vi "DAQ Loop.vi"(7 "DAQ Exit":refnum<notifier>, 8 "error in":errorcluster, 10 "DAQ Queue":refnum<queue>, 11 "PLC Queue":refnum<queue>) -> (0 "error out":errorcluster)   [LabVIEW 2014, in "DAQ.lvlib"]
uses:
  DAQ.lvlib
  support/Message Queue/Message Queue.lvlib
  <vilib>/Utility/error.llb/Error Cluster From Error Code.vi
  support/Message Queue/Enqueue Message (Single).vi
  TypeDefs/DAQ data.ctl
  <vilib>/ErrorRing/Error Ring.xnode
  support/Message Queue/Message Cluster.ctl
panel:
  out "DAQ message":string
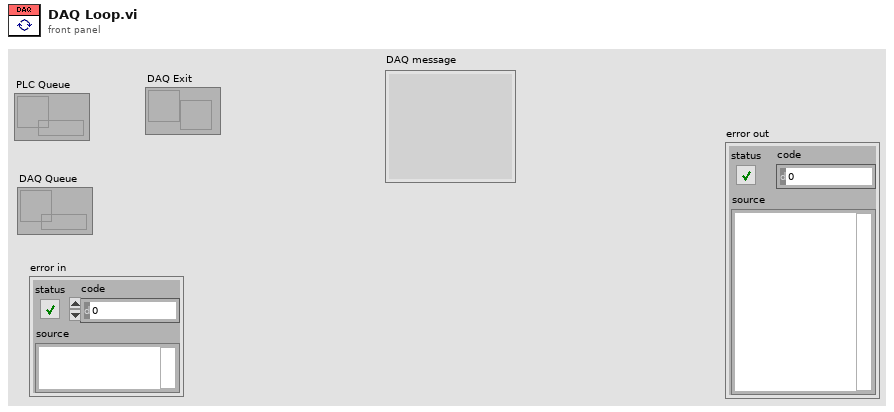
[diagram p1: front panel]
types:
  T1 = typedef "DAQ.lvlib/DAQ data.ctl" = cluster{"Power switch (DI)":cluster{"Channel":tag, "Data":bool}, "Dispose barrel (DI)":cluster{"Channel":tag, "Data":bool}, "Pump status (DO)":cluster{"Channel":tag, "Data":bool}, "Barrel position (AI)":cluster{"Channel":tag, "Data":dbl}}
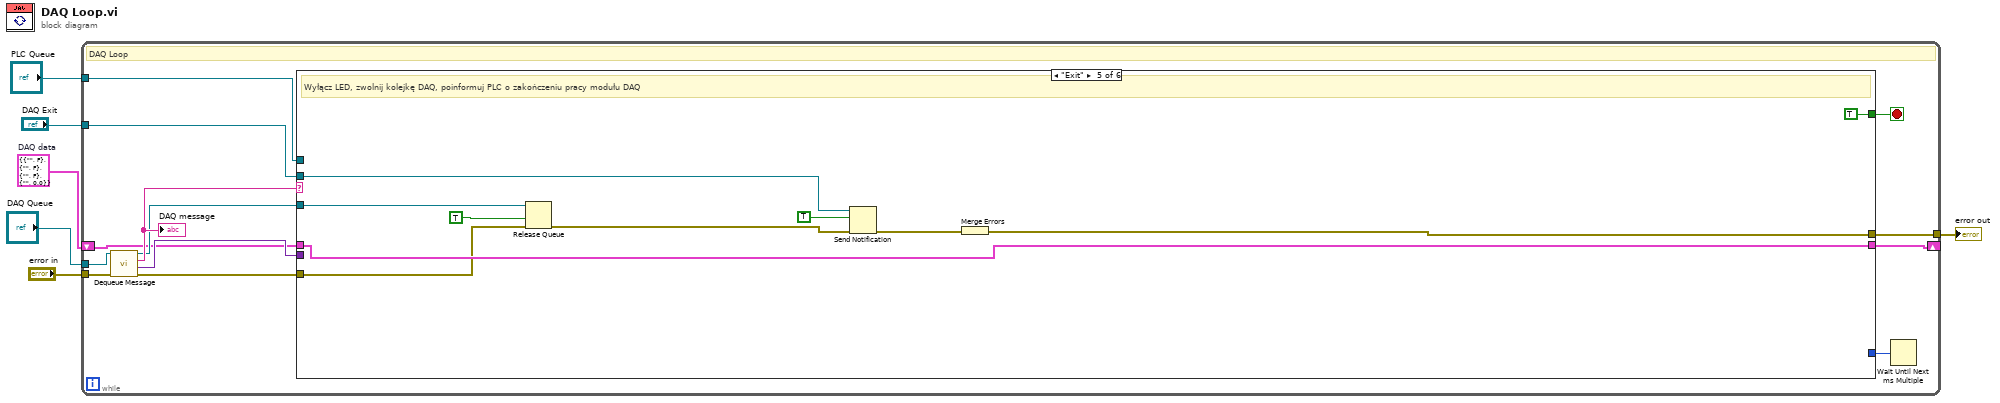
[diagram p0: block diagram]
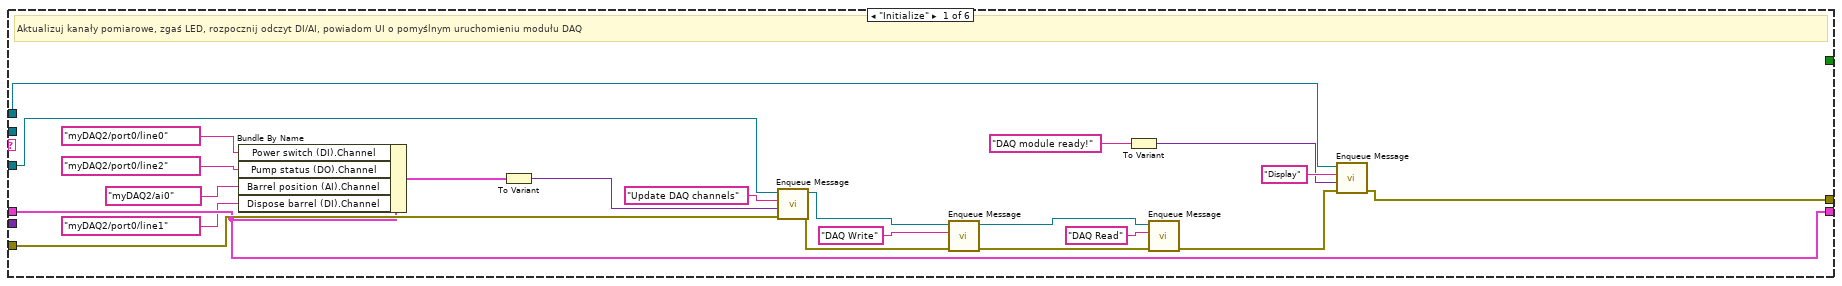
[diagram p2: hidden frame]
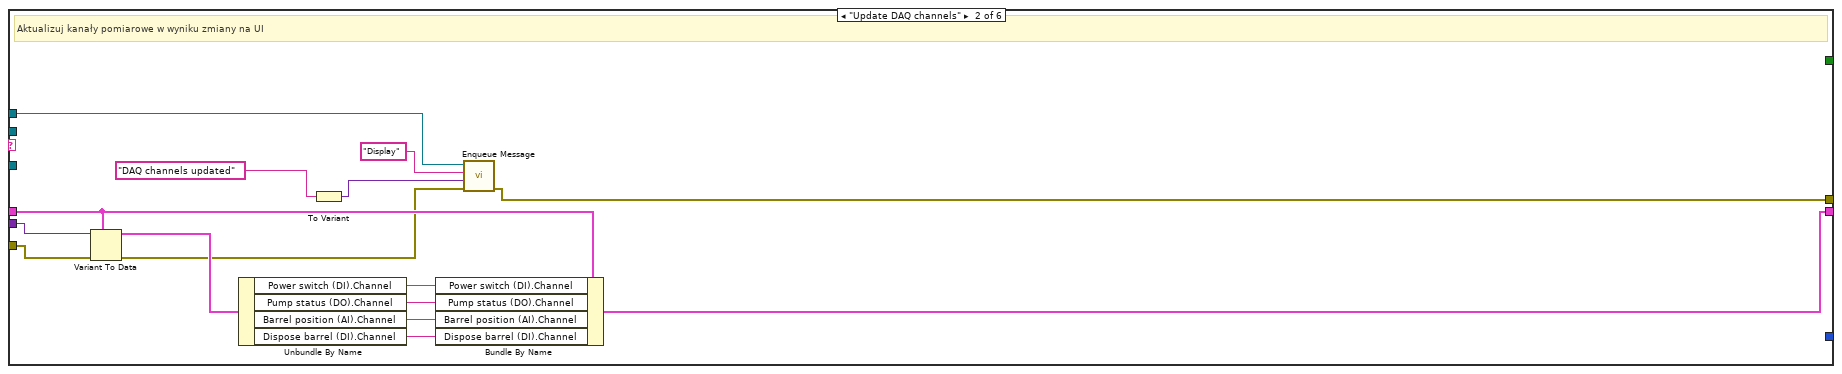
[diagram p3: hidden frame]
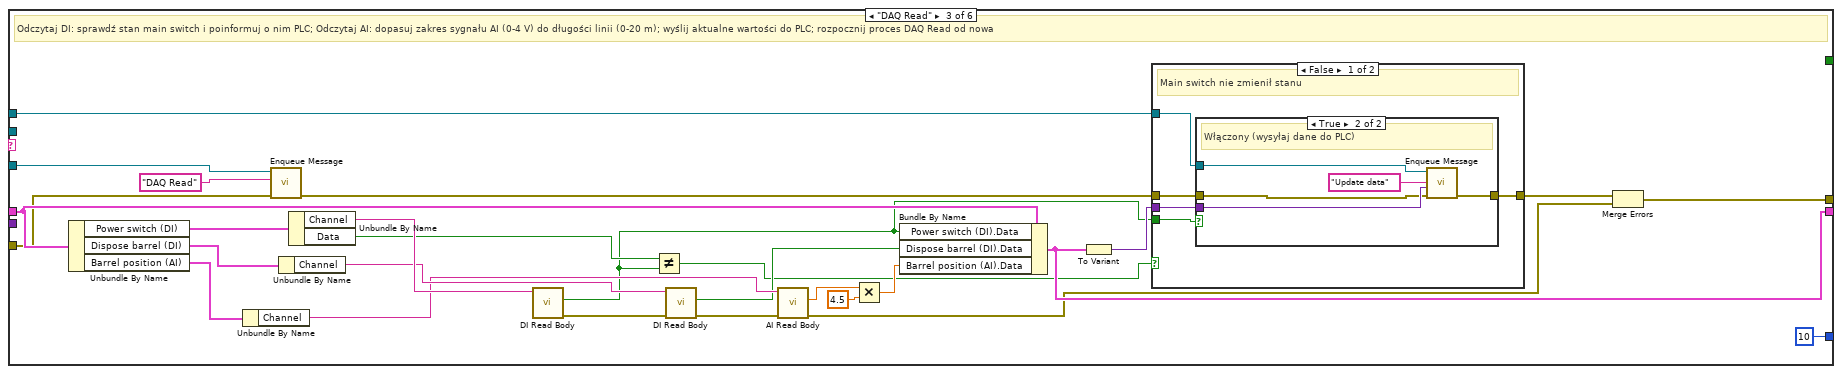
[diagram p4: hidden frame]
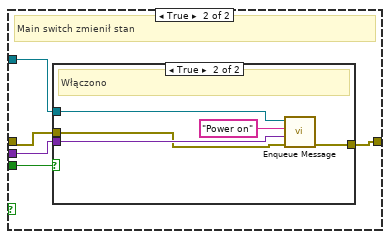
[diagram p6: hidden frame]
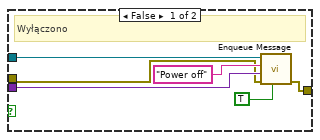
[diagram p7: hidden frame]
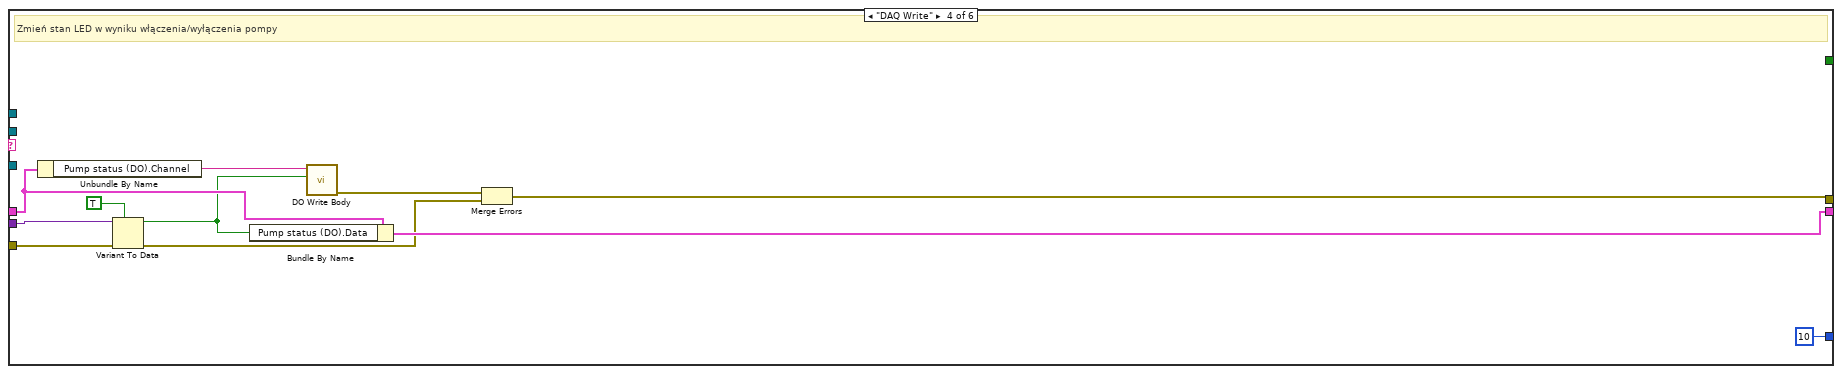
[diagram p8: hidden frame]
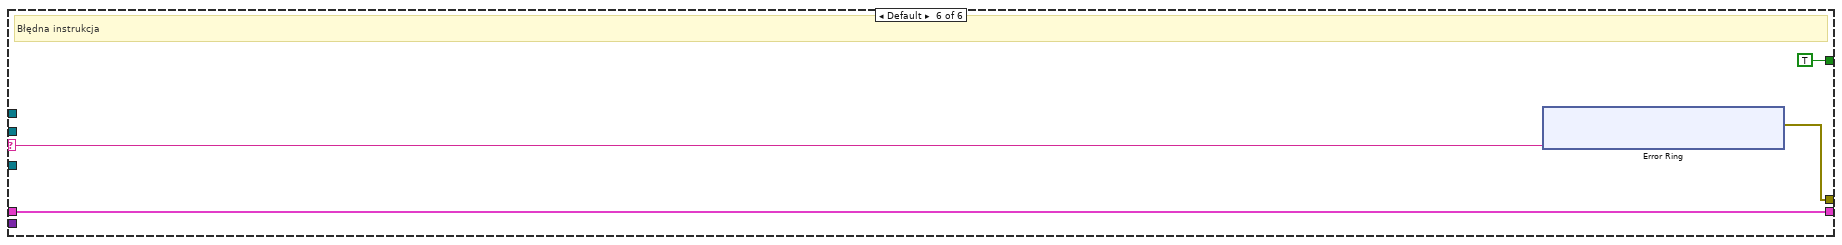
[diagram p9: hidden frame]
diagram:
  w5 = T1 {"Power switch (DI)"={"Channel"="", "Data"=FALSE}, "Dispose barrel (DI)"={"Channel"="", "Data"=FALSE}, "Pump status (DO)"={"Channel"="", "Data"=FALSE}, "Barrel position (AI)"={"Channel"="", "Data"=0.0}}  # DAQ data
  n1 = while {
    tunnel: "error in" -> [w18]
    tunnel: "DAQ Queue" -> [w13]
    tunnel: [w16] -> w2
    tunnel: "PLC Queue" -> [w12]
    tunnel: "DAQ Exit" -> [w10]
    shift-right: [w8] -> _
    shift-left: w5 -> [w9]
    stop <- w14 stop-if-true
    # "DAQ Loop"
    n2 = call "Dequeue Message.vi"("error in (no error)"=w18, "Message Queue"=w13) -> ("error out"=w17:errorcluster, "Message Data"=w15:variant, "Message"=w19:string, "dup Message Queue"=w11:refnum<queue>)  [unwired: 6 in]
    "DAQ message" <- w19
    n3 = case shown="\"Exit\"" w19 {
      selector: w19 -> [_ _ _ _ _ w133]
      tunnel: w17 -> [w38 w55 w60 w120 w123 _]
      tunnel: [w35 w45 w57 w111 w122 w132] -> w16
      tunnel: w15 -> [_ w56 _ w119 _ _]
      tunnel: w12 -> [w39 w44 w65 _ _ _]
      tunnel: [_ _ _ _ TRUE TRUE] -> w14
      tunnel: w11 -> [w37 _ w77 _ w131 _]
      tunnel: w10 -> [_ _ _ _ w130 _]
      tunnel: w9 -> [w27 w53 w78 w116 w125 w134]
      tunnel: [w27 w48 w68 w118 w125 w134] -> w8
      tunnel: [_ _ u32 10 ("millisecond multiple") u32 10 ("millisecond multiple") _ _] -> w7
      frame "Initialize" {
        # "Aktualizuj kanały pomiarowe, zgaś LED, rozpocznij odczyt DI/AI, powiadom UI o pomyślnym uruchomieniu modułu DAQ"
        n4 = Bundle By Name(cluster=w27, "Power switch (DI).Channel"=tag "myDAQ2/port0/line0", "Pump status (DO).Channel"=tag "myDAQ2/port0/line2" ("Power switch (DI).Channel"), "Barrel position (AI).Channel"=tag "myDAQ2/ai0", "Dispose barrel (DI).Channel"=tag "myDAQ2/port0/line1" ("Power switch (DI).Channel")) -> (w26:T1)
        n5 = To Variant(anything=w26) -> (Variant=w25:variant)
        n6 = call-poly "Enqueue Message.vi"("error in (no error)"=w38, "Message Data"=w25, "Message"="Update DAQ channels", "Message Queue"=w37) -> ("error out"=w32:errorcluster, "dup Message Queue"=w31:refnum<queue>)  [unwired: 6 in]
        n7 = call-poly "Enqueue Message.vi"("error in (no error)"=w32, "Message"="DAQ Write", "Message Queue"=w31) -> ("error out"=w29:errorcluster, "dup Message Queue"=w28:refnum<queue>)  [unwired: 7 in]
        n8 = To Variant(anything="DAQ module ready!" ("Message")) -> (Variant=w20:variant)
        n9 = call-poly "Enqueue Message.vi"("error in (no error)"=w29, "Message"="DAQ Read", "Message Queue"=w28) -> ("error out"=w34:errorcluster)  [unwired: 7 in, 1 out]
        n10 = call-poly "Enqueue Message.vi"("error in (no error)"=w34, "Message Data"=w20, "Message"="Display", "Message Queue"=w39) -> ("error out"=w35:errorcluster)  [unwired: 6 in, 1 out]
      }
      frame "Update DAQ channels" {
        # "Aktualizuj kanały pomiarowe w wyniku zmiany na UI"
        n11 = Variant To Data(error in=w55, type=w53, Variant=w56) -> (data=w54:T1, error out=w46:errorcluster)
        n12 = Unbundle By Name(w54) -> ("Power switch (DI).Channel"=w52:tag, "Pump status (DO).Channel"=w51:tag, "Barrel position (AI).Channel"=w50:tag, "Dispose barrel (DI).Channel"=w49:tag)
        n13 = To Variant(anything="DAQ channels updated" ("Message")) -> (Variant=w42:variant)
        n14 = Bundle By Name(cluster=w53, "Power switch (DI).Channel"=w52, "Pump status (DO).Channel"=w51, "Barrel position (AI).Channel"=w50, "Dispose barrel (DI).Channel"=w49) -> (w48:T1)
        n15 = call-poly "Enqueue Message.vi"("error in (no error)"=w46, "Message Data"=w42, "Message"="Display", "Message Queue"=w44) -> ("error out"=w45:errorcluster)  [unwired: 6 in, 1 out]
      }
      frame "DAQ Read" {
        # "Odczytaj DI: sprawdź stan main switch i poinformuj o nim PLC; Odczytaj AI: dopasuj zakres sygnału AI (0-4 V) do długości linii (0-20 m); wyślij aktualne wartości do PLC; rozpocznij proces DAQ Read od nowa"
        n16 = Unbundle By Name(w78) -> ("Power switch (DI)"=w76:cluster{"Channel":tag, "Data":bool}, "Dispose barrel (DI)"=w74:cluster{"Channel":tag, "Data":bool}, "Barrel position (AI)"=w72:cluster{"Channel":tag, "Data":dbl})
        n17 = Unbundle By Name(w72) -> ("Channel"=w71:tag)
        n18 = call-poly "Enqueue Message.vi"("error in (no error)"=w60, "Message"="DAQ Read", "Message Queue"=w77) -> ("error out"=w58:errorcluster)  [unwired: 7 in, 1 out]
        n19 = Unbundle By Name(w74) -> ("Channel"=w73:tag)
        n20 = Unbundle By Name(w76) -> ("Channel"=w75:tag, "Data"=w67:bool)
        n21 = call "DI Read Body.vi"("Channel"=w75) -> ("error out"=w83:errorcluster, "data"=w62:bool)  [unwired: 7 in]
        n22 = Not Equal?(x=w67, y=w62) -> (x != y?=w63:bool)
        n23 = call "DI Read Body.vi"("error in"=w83, "Channel"=w73) -> ("error out"=w82:errorcluster, "data"=w66:bool)  [unwired: 6 in]
        n24 = call "AI Read Body.vi"("error in"=w82, "Channel"=w71) -> ("error out"=w61:errorcluster, "data"=w80:dbl)  [unwired: 6 in]
        n25 = Multiply(x=w80, y=4.5) -> (x*y=w70:dbl)
        n26 = Bundle By Name(cluster=w78, "Power switch (DI).Data"=w62, "Dispose barrel (DI).Data"=w66, "Barrel position (AI).Data"=w70) -> (w68:T1)
        n27 = To Variant(anything=w68) -> (Variant=w64:variant)
        n28 = case shown="False" w63 {
          tunnel: w65 -> [w86 w99]
          tunnel: w64 -> [w88 w98]
          tunnel: [w87 w97] -> w59
          tunnel: w62 -> [w85 w96]
          tunnel: w58 -> [w84 w95]
          frame False {
            # "Main switch nie zmienił stanu"
            n29 = case shown="True" w85 {
              tunnel: w86 -> [_ w94]
              tunnel: w88 -> [_ w93]
              tunnel: [w89 w92] -> w87
              tunnel: w84 -> [w89 w90]
              frame False {
                # "Wyłączony"
              }
              frame True {
                # "Włączony (wysyłaj dane do PLC)"
                n30 = call-poly "Enqueue Message.vi"("error in (no error)"=w90, "Message Data"=w93, "Message"="Update data", "Message Queue"=w94) -> ("error out"=w92:errorcluster)  [unwired: 6 in, 1 out]
              }
            }
          }
          frame True {
            # "Main switch zmienił stan"
            n31 = case shown="True" w96 {
              tunnel: w99 -> [w105 w110]
              tunnel: w98 -> [w104 w109]
              tunnel: [w103 w108] -> w97
              tunnel: w95 -> [w100 w106]
              frame False {
                # "Wyłączono"
                n32 = call-poly "Enqueue Message.vi"("Priority Message? (F)"=TRUE, "error in (no error)"=w100, "Message Data"=w104, "Message"="Power off", "Message Queue"=w105) -> ("error out"=w103:errorcluster)  [unwired: 5 in, 1 out]
              }
              frame True {
                # "Włączono"
                n33 = call-poly "Enqueue Message.vi"("error in (no error)"=w106, "Message Data"=w109, "Message"="Power on", "Message Queue"=w110) -> ("error out"=w108:errorcluster)  [unwired: 6 in, 1 out]
              }
            }
          }
        }
        n34 = Merge Errors(w59, w61) -> (w57:errorcluster)
      }
      frame "DAQ Write" {
        # "Zmień stan LED w wyniku włączenia/wyłączenia pompy"
        n35 = Unbundle By Name(w116) -> ("Pump status (DO).Channel"=w117:tag)
        n36 = Variant To Data(error in=w120, type=TRUE, Variant=w119) -> (data=w114:bool, error out=w112:errorcluster)
        n37 = Bundle By Name(cluster=w116, "Pump status (DO).Data"=w114) -> (w118:T1)
        n38 = call "DO Write Body.vi"("data"=w114, "Channel"=w117) -> ("error out"=w113:errorcluster)  [unwired: 7 in]
        n39 = Merge Errors(w113, w112) -> (w111:errorcluster)
      }
      frame "Exit" {
        # "Wyłącz LED, zwolnij kolejkę DAQ, poinformuj PLC o zakończeniu pracy modułu DAQ"
        n40 = Release Queue(queue=w131, force destroy? (F)=TRUE, error in (no error)=w123) -> (error out=w128:errorcluster)  [unwired: 2 out]
        n41 = Send Notification(notification=TRUE, notifier=w130, error in (no error)=w128) -> (error out=w124:errorcluster)  [unwired: 1 out]
        n42 = Merge Errors(w124) -> (w122:errorcluster)
      }
      frame Default {
        # "Błędna instrukcja"
        n43 = xnode "Error Ring"("parameter 0"=w133) -> ("error out"=w132:errorcluster)
      }
    }
    n44 = Wait Until Next ms Multiple(millisecond multiple=w7) -> ()  [unwired: 1 out]
  }
  "error out" <- w2
